vi "pmu_Create Time Queue.vi"(8 "error in (no error)":errorcluster, 11 "PMU System Info in":refnum<class "PMU System Info.lvclass">) -> (0 "error out":errorcluster, 3 "PMU System Info out":refnum<class "PMU System Info.lvclass">)   [LabVIEW 2011, in "NI_EP_PMU.lvlib" / "PMU System Info.lvclass"]
uses:
  <vilib>/addons/Electrical Power/PMU/Common/Classes/PMU System Info/PMU System Info.lvclass
  <vilib>/addons/Electrical Power/PMU/Common/Controls/pmu_Time&Quality.ctl
  <vilib>/addons/Electrical Power/PMU/Common/Classes/PMU System Info/PMU System Info.lvclass/PMU System Info.ctl
  <vilib>/addons/Electrical Power/PMU/NI_EP_PMU.lvlib
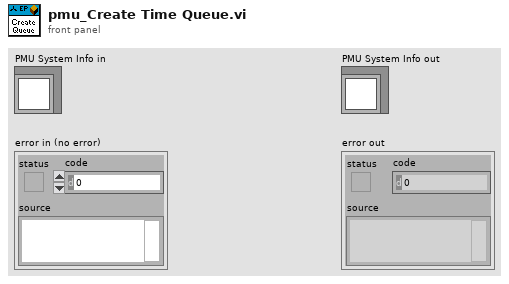
[diagram p1: front panel]
types:
  T1 = typedef "NI_EP_PMU.lvlib/pmu_Time&Quality.ctl" = cluster{"time stamp":timestamp, "time quality":u8}
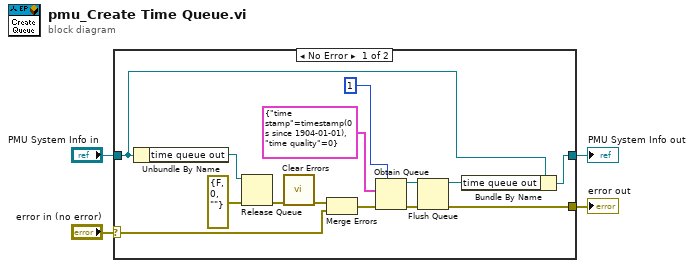
[diagram p0: block diagram]
diagram:
  n1 = case shown="No Error" "error in (no error)" {
    selector: "error in (no error)" -> [w6 w19]
    tunnel: [w14 w19] -> w1
    tunnel: "PMU System Info in" -> [w12 w20]
    tunnel: [w15 w20] -> w2
    frame No Error {
      n2 = Unbundle By Name(w12) -> ("time queue out"=w11:refnum<queue>)
      n3 = Release Queue(queue=w11, error in (no error)=errorcluster {"status"=FALSE, "code"=0, "source"=""}) -> (error out=w9:errorcluster)  [unwired: 1 in, 2 out]
      n4 = call <vilib>:"Clear Errors.vi"("error in (no error)"=w9) -> ("error out"=w7:errorcluster)  [unwired: 6 in]
      n5 = Merge Errors(w7, w6) -> (w5:errorcluster)
      n6 = Obtain Queue(max queue size (-1, unlimited)=1, element data type=T1 {"time stamp"=timestamp(0 s since 1904-01-01), "time quality"=0} ("Time"), error in (no error)=w5) -> (queue out=w10:refnum<queue>, error out=w17:errorcluster)  [unwired: 2 in, 1 out]
      n7 = Flush Queue(queue=w10, error in (no error)=w17) -> (queue out=w16:refnum<queue>, error out=w14:errorcluster)  [unwired: 1 out]
      n8 = Bundle By Name(cluster=w12, "time queue out"=w16) -> (w15:refnum<class "PMU System Info.lvclass">)
    }
    frame Error {
    }
  }
  "error out" <- w1
  "PMU System Info out" <- w2
